vi "export_avg_traj.vi"(0 "file name":string="avg_trajectory.csv", 1 "BoundaryZpelv":dbl[](array[numeric]), 2 "BoundaryYpelv":dbl[](array[numeric]), 3 "BoundaryXpelv":dbl[](array[numeric]), 4 "Host folder":path=path "C:/Users/User/Documents/GitHub/RobUST/Labview/RobUST_3D/Recorded Data") -> ()   [LabVIEW 2024]
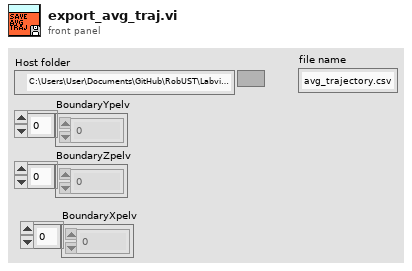
[diagram p1: front panel]
types:
  T1 = enum16{"open", "replace", "create", "open or create", "replace or create", "replace or create with confirmation"}
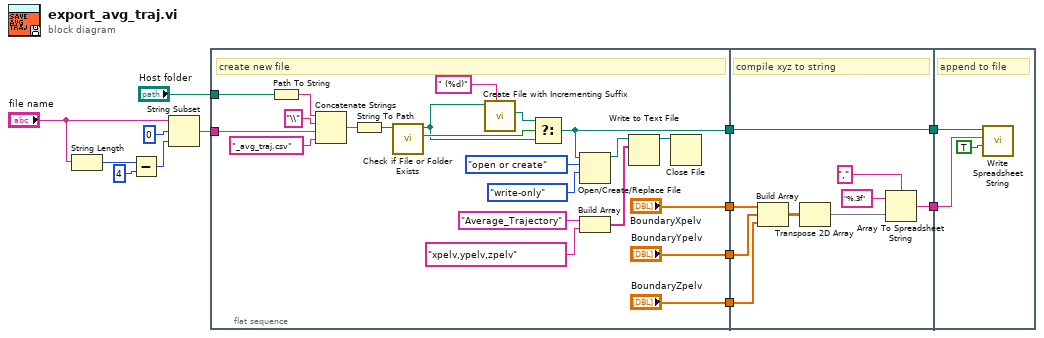
[diagram p0: block diagram]
diagram:
  n1 = String Length(string="file name") -> (length=w3:i32)
  n2 = Subtract(x=w3, y=4) -> (x-y=w1:i32)
  n3 = String Subset(string="file name", offset (0)=0, length (rest)=w1) -> (substring=w6:string)
  n4 = flat-sequence {
    tunnel: "Host folder" -> [w27]
    tunnel: w6 -> [w20]
    tunnel: [w23] -> w13
    tunnel: ["BoundaryXpelv"] -> w11
    tunnel: ["BoundaryYpelv"] -> w10
    tunnel: ["BoundaryZpelv"] -> w9
    tunnel: w13 -> [w44]
    tunnel: w11 -> [w40]
    tunnel: w10 -> [w39]
    tunnel: w9 -> [w38]
    tunnel: [w44] -> w8
    tunnel: [w41] -> w7
    tunnel: w8 -> [w46]
    tunnel: w7 -> [w47]
    frame #0 {
      # "create new file"
      n5 = Path To String(path=w27) -> (string=w32:string)
      n6 = Concatenate Strings(w32, "\\" ("string"), w20, "_avg_traj.csv" ("string")) -> (w31:string)
      n7 = String To Path(string=w31) -> (path=w34:path)
      n8 = call <vilib>:"Check if File or Folder Exists.vi"("path"=w34) -> ("file or folder exists?"=w35:bool, "dup path"=w30:path)  [unwired: 8 in, 1 out]
      n9 = call <vilib>:"Create File with Incrementing Suffix.vi"("format string (\" (%d)\")"=" (%d)" ("format string (\" (%d)\")"), "file path"=w30) -> ("actual path"=w29:path)  [unwired: 7 in, 2 out]
      n10 = Select(t=w29, s=w35, f=w30) -> (s? t:f=w23:path)
      n11 = Open/Create/Replace File(file path (use dialog)=w23, operation (0:open)=T1."open or create", access (0:read/write)=enum16{"read/write", "read-only", "write-only"}."write-only") -> (refnum out=w24:refnum<file>)  [unwired: 3 in, 2 out]
      n12 = Build Array("Average_Trajectory" ("element"), "xpelv,ypelv,zpelv" ("String")) -> (w21:string[])
      n13 = Write to Text File(file (use dialog)=w24, text=w21) -> (refnum out=w22:refnum<file>)  [unwired: 2 in, 2 out]
      n14 = Close File(refnum=w22) -> ()  [unwired: 1 in, 2 out]
    }
    frame #1 {
      # "compile xyz to string"
      n15 = Build Array(w40, w39, w38) -> (w37:dbl[][])
      n16 = Transpose 2D Array(2D array=w37) -> (transposed array=w36:dbl[][])
      n17 = Array To Spreadsheet String(delimiter (Tab)="," ("delimiter (\\t)"), array=w36, 3:"%.3f" ("format string")) -> (spreadsheet string=w41:string)
    }
    frame #2 {
      # "append to file"
      n18 = call <vilib>:"Write Spreadsheet String.vi"("append to file? (new file:F)"=TRUE, "spreadsheet string"=w47, "file path (dialog if empty)"=w46) -> ()  [unwired: 7 in, 2 out]
    }
  }
